vi "test Import Messages.vi"(8 "error in":errorcluster, 11 "TestCase in":refnum<class "1553 Parameters Import.lvclass">) -> (0 "error out":errorcluster, 3 "TestCase out":refnum<class "1553 Parameters Import.lvclass">)   [LabVIEW 2020, in "1553 Parameters Import.lvclass"]
uses:
  1553 Parameters Import.lvclass
  Shared/Message Definition.ctl
  Shared/Message Type.ctl
  Shared/Terminal Endpoint.ctl
  Shared/Address.ctl
  Shared/Parameter Definition.ctl
  1553 Parameters Import.lvclass/1553 Parameters Import.ctl
  <vilib>/addons/_JKI Toolkits/VI Tester/TestCase.llb/TestCase.lvclass
  C:/Program Files (x86)/National Instruments/LabVIEW 2020/vi.lib/addons/_JKI Toolkits/VI Tester/TestCase.llb/TestCase.lvclass
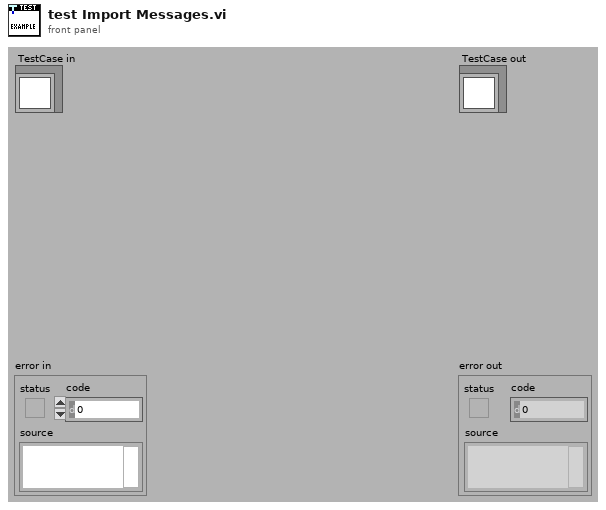
[diagram p1: front panel]
types:
  T1 = typedef "Message Definition.ctl" = cluster{"name":string, "message type":T2, "endpoint Rx":T3, "endpoint Tx":T3, "mode code":u16, "number of words":u16, "parameters":cluster{"name":string, "default value":dbl, "unit":string, "parameter definition":T5}[], "create timestamp channel":bool}
  T2 = typedef "Message Type.ctl" = string
  T3 = typedef "Terminal Endpoint.ctl" = cluster{"terminal address":T4, "subaddress":T4}
  T4 = typedef "Address.ctl" = u16
  T5 = typedef "Parameter Definition.ctl" = cluster{"start index":i32, "size (bits)":i32, "encoding":enum16{"BNR", "BCD", "Discrete"}, "signed":bool, "multiplier":dbl, "offset":dbl}
  T6 = typedef "1553 Channel.ctl" = cluster{"HW channel":u16, "terminals":T7[], "messages":T1[], "acyclic frame names":string[]}
  T7 = typedef "Terminal Name and Address.ctl" = cluster{"name":string, "terminal address":T4}
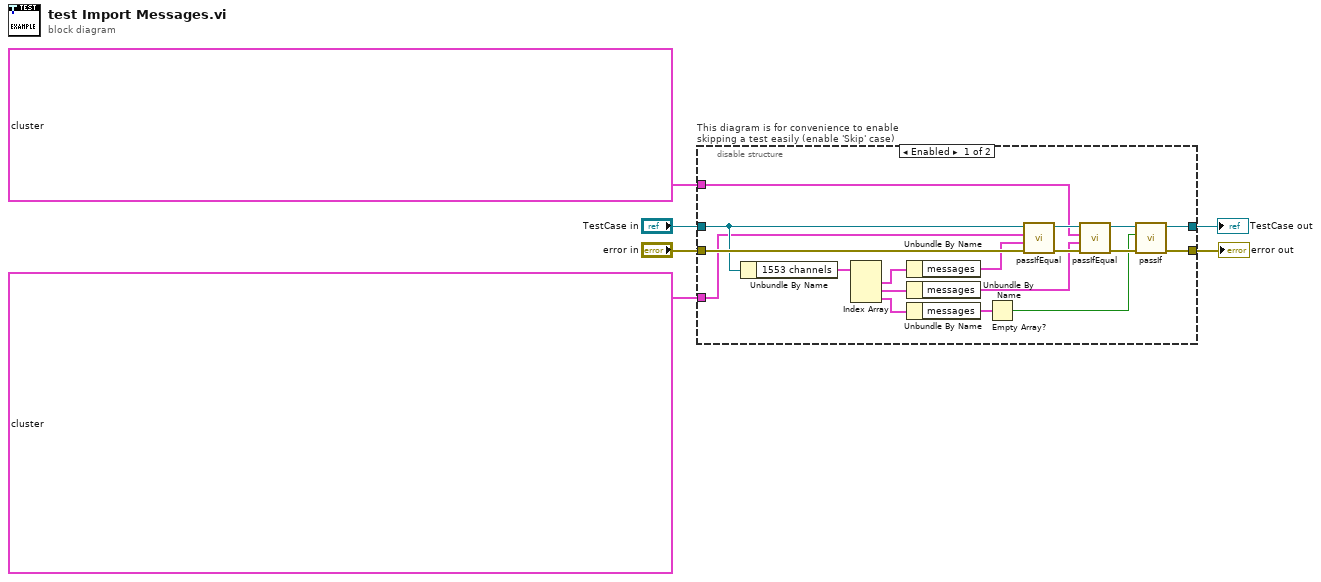
[diagram p0: block diagram]
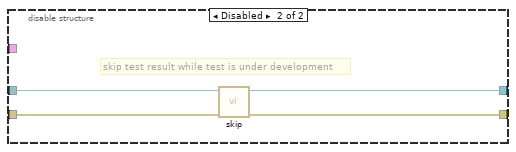
[diagram p2: hidden frame]
diagram:
  n1 = disable-structure "This diagram is for convenience to enable skipping a test easily (enable 'Skip' case)" shown="Enabled" {
    disable-tunnel: "TestCase in" -> [w12 w28]
    disable-tunnel: [w17 w26] -> w3
    disable-tunnel: [w18 w27] -> w5
    disable-tunnel: "error in" -> [w13 w25]
    disable-tunnel: T1[] [{"name"="Latitude", "message type"="BC to RT", "endpoint Rx"={"terminal address"=21, "subaddress"=7}, "endpoint Tx"={"terminal address"=0, "subaddress"=0}, "mode code"=0, "number of words"=3, "parameters"=[{"name"="Parameter 0", "default value"=0.0, "unit"="deg", "parameter definition"={"start index"=16, "size (bits)"=32, "encoding"=enum."BNR", "signed"=TRUE, "multiplier"=3600.0, "offset"=0.0}}], "create timestamp channel"=TRUE}, {"name"="Longitude", "message type"="RT to BC", "endpoint Rx"={"terminal address"=0, "subaddress"=0}, "endpoint Tx"={"terminal address"=22, "subaddress"=7}, "mode code"=0, "number of words"=3, "parameters"=[{"name"="Parameter 0", "default value"=0.0, "unit"="deg", "parameter definition"={"start index"=16, "size (bits)"=32, "encoding"=enum."BNR", "signed"=TRUE, "multiplier"=3600.0, "offset"=0.0}}], "create timestamp channel"=TRUE}, {"name"="Position", "message type"="RT to RT", "endpoint Rx"={"terminal address"=11, "subaddress"=12}, "endpoint Tx"={"terminal address"=1, "subaddress"=2}, "mode code"=0, "number of words"=6, "parameters"=[{"name"="Latitude", "default value"=0.0, "unit"="deg", "parameter definition"={"start index"=16, "size (bits)"=32, "encoding"=enum."BNR", "signed"=TRUE, "multiplier"=360000.0, "offset"=0.0}}, {"name"="Longitude", "default value"=0.0, "unit"="deg", "parameter definition"={"start index"=64, "size (bits)"=32, "encoding"=enum."BNR", "signed"=TRUE, "multiplier"=360000.0, "offset"=0.0}}], "create timestamp channel"=FALSE}] ("messages") -> [w8 _]
    disable-tunnel: T1[] [{"name"="Position", "message type"="RT to RT", "endpoint Rx"={"terminal address"=11, "subaddress"=12}, "endpoint Tx"={"terminal address"=1, "subaddress"=2}, "mode code"=0, "number of words"=6, "parameters"=[{"name"="Word 00", "default value"=1.0, "unit"="", "parameter definition"={"start index"=0, "size (bits)"=16, "encoding"=enum."BNR", "signed"=FALSE, "multiplier"=1.0, "offset"=0.0}}, {"name"="Word 01", "default value"=1.0, "unit"="", "parameter definition"={"start index"=16, "size (bits)"=16, "encoding"=enum."BNR", "signed"=FALSE, "multiplier"=1.0, "offset"=0.0}}, {"name"="Word 02", "default value"=1.0, "unit"="", "parameter definition"={"start index"=32, "size (bits)"=16, "encoding"=enum."BNR", "signed"=FALSE, "multiplier"=1.0, "offset"=0.0}}, {"name"="Word 03", "default value"=1.0, "unit"="", "parameter definition"={"start index"=48, "size (bits)"=16, "encoding"=enum."BNR", "signed"=FALSE, "multiplier"=1.0, "offset"=0.0}}, {"name"="Word 04", "default value"=1.0, "unit"="", "parameter definition"={"start index"=64, "size (bits)"=16, "encoding"=enum."BNR", "signed"=FALSE, "multiplier"=1.0, "offset"=0.0}}, {"name"="Word 05", "default value"=1.0, "unit"="", "parameter definition"={"start index"=80, "size (bits)"=16, "encoding"=enum."BNR", "signed"=FALSE, "multiplier"=1.0, "offset"=0.0}}], "create timestamp channel"=TRUE}] ("messages") -> [w7 _]
    frame Enabled {
      n2 = Unbundle By Name(w12) -> ("1553 channels"=w11:T6[])
      n3 = Index Array(array=w11) -> (element #1=w24:T6, element #2=w22:T6, element #3=w16:T6)  [unwired: 3 in]
      n4 = Unbundle By Name(w24) -> ("messages"=w10:T1[])
      n5 = Unbundle By Name(w22) -> ("messages"=w9:T1[])
      n6 = Unbundle By Name(w16) -> ("messages"=w15:T1[])
      n7 = Empty Array?(array=w15) -> (empty?=w14:bool)
      n8 = call-dynamic "passIfEqual.vi"("error in (no error)"=w13, "y"=w10, "x"=w8, "TestCase in"=w12) -> ("error out"=w23:errorcluster, "TestCase out"=w21:refnum<class "1553 Parameters Import.lvclass">)  [unwired: 6 in]
      n9 = call-dynamic "passIfEqual.vi"("error in (no error)"=w23, "y"=w9, "x"=w7, "TestCase in"=w21) -> ("error out"=w20:errorcluster, "TestCase out"=w19:refnum<class "1553 Parameters Import.lvclass">)  [unwired: 6 in]
      n10 = call-dynamic "passIf.vi"("error in (no error)"=w20, "pass"=w14, "TestCase in"=w19) -> ("error out"=w18:errorcluster, "TestCase out"=w17:refnum<class "1553 Parameters Import.lvclass">)  [unwired: 7 in]
    }
    frame Disabled {
      # "skip test result while test is under development"
      n11 = call <vilib>:"skip.vi"("error in (no error)"=w25, "TestCase in"=w28) -> ("error out"=w27:errorcluster, "TestCase out"=w26:refnum<class "1553 Parameters Import.lvclass">)  [unwired: 8 in]
    }
  }
  "error out" <- w5
  "TestCase out" <- w3
